vi "10 to 16.vi"(10 "字符串":string) -> (2 "字符串 2":string)   [LabVIEW 2021]
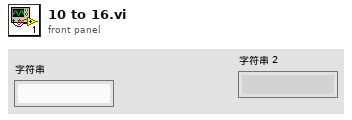
[diagram p1: front panel]
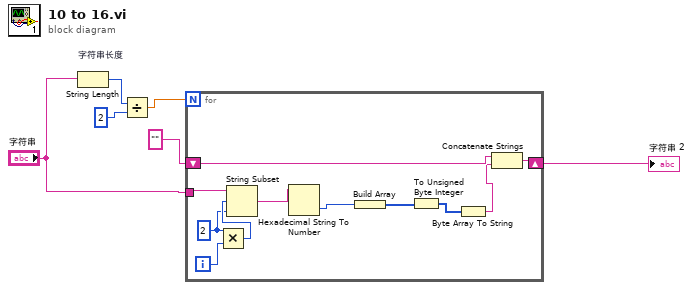
[diagram p0: block diagram]
diagram:
  n1 = String Length "字符串长度"(string="字符串") -> (length=w6:i32)
  n2 = Divide(x=w6, y=2) -> (x/y=w4:dbl)
  n3 = for {
    N: w4 -> [_]
    shift-right: [w15] -> w1
    shift-left: "" -> [w16]
    tunnel: "字符串" -> [w14]
    i -> [w13]
    w11 = 2
    n4 = Multiply(x=w11, y=w13) -> (x*y=w12:i32)
    n5 = String Subset(string=w14, offset (0)=w12, length (rest)=w11) -> (substring=w17:string)
    n6 = Hexadecimal String To Number(string=w17) -> (number=w10:u32)  [unwired: 2 in, 1 out]
    n7 = Build Array(w10) -> (w9:u32[])
    n8 = To Unsigned Byte Integer(number=w9) -> (unsigned 8bit integer=w8:u8[])
    n9 = Byte Array To String(unsigned byte array=w8) -> (string=w7:string)
    n10 = Concatenate Strings(w16, w7) -> (w15:string)
  }
  "字符串 2" <- w1
